vi "SSD1306_SaveFonts2File.vi"(1 "vi name":string) -> (0 "file name":string)   [LabVIEW 2014, in "QwaveSys_Interface.lvlib"]
uses:
  QwaveSys_Interface.lvlib
  <vilib>/Utility/traverseref.llb/TRef TravTarget.ctl
  <vilib>/Utility/sysdir.llb/System Directory Type.ctl
  <vilib>/Utility/traverseref.llb/VI Scripting - Traverse.lvlib
panel:
  out "error out":errorcluster
  out "found":bool
  out "Fonts":string
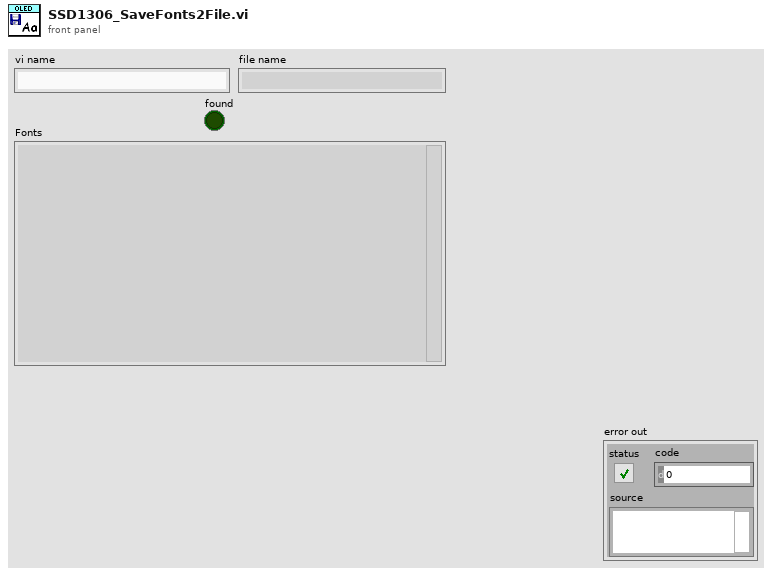
[diagram p1: front panel]
types:
  T1 = typedef "System Directory Type.ctl" = i32
  T2 = typedef "TRef TravTarget.ctl" = enum16{"FP", "BD", "Other"}
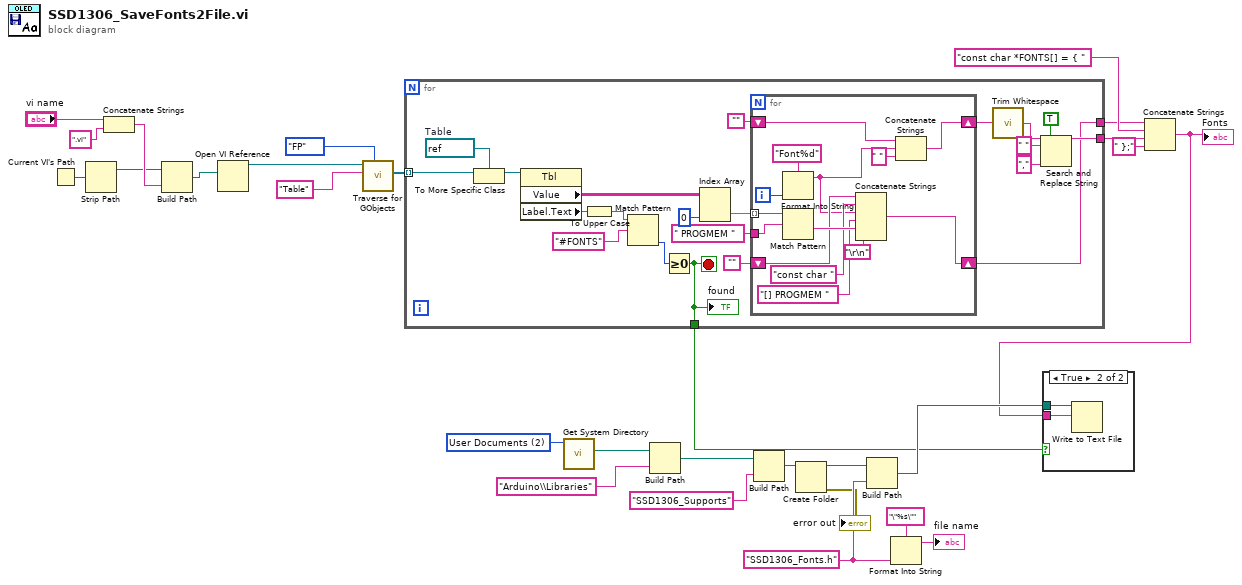
[diagram p0: block diagram]
diagram:
  w18 = T1 2 items=["User Home"=0, "User Desktop"=1, "User Documents"=2, "User Application Data"=3, "User Preferences"=4, "User Temporary"=5, "Public Documents"=6, "Public Application Data"=7, "Public Preferences"=8, "Public Cache"=13, "System Core Libraries"=9, "System Installed Libraries"=10, "Application Files"=11, "Boot Volume Root"=12] ("system directory type")
  w13 = "SSD1306_Fonts.h" ("string")
  n1 = Current VI's Path() -> (path=w22:path)
  n2 = Strip Path(path=w22) -> (stripped path=w21:path)  [unwired: 1 out]
  n3 = Concatenate Strings("vi name", ".vi" ("string")) -> (w23:string)
  n4 = Build Path(base path=w21, name or relative path=w23) -> (appended path=w19:path)
  n5 = Open VI Reference(vi path=w19) -> (vi reference=w28:refnum<vi>)  [unwired: 5 in, 1 out]
  n6 = call <vilib>:"Traverse for GObjects.vi"("Traverse Target"=TRef_TravTarget."FP", "Class Name"="Table", "VI Refnum"=w28) -> ("References"=w26:refnum<vi>[])  [unwired: 5 in, 3 out]
  n7 = for {
    tunnel: w26 -> [w48] mode=indexing
    tunnel: [w37] -> w8
    tunnel: [w31] -> w6
    tunnel: [w29] -> w3
    stop <- w37 stop-if-true
    w47 = refnum<vi> refnum  # Table
    n8 = To More Specific Class(target class=w47, reference=w48) -> (specific class reference=w49:refnum<vi>)  [unwired: 1 in, 1 out]
    n9 = property class="Tbl"(reference=w49) -> ("Value"=w42:string[][], "Label.Text"=w46:string)  [unwired: 1 in, 2 out]
    n10 = To Upper Case(1:w46) -> (0:w45:string)
    n11 = Match Pattern(string=w45, regular expression="#FONTS") -> (offset past match=w44:i32)  [unwired: 1 in, 3 out]
    n12 = Greater Or Equal To 0?(x=w44) -> (x >= 0?=w37:bool)
    "found" <- w37
    n13 = Index Array(array=w42, index (col)=0 ("disabled index (col)")) -> (element=w40:string[])  [unwired: 1 in]
    n14 = for {
      tunnel: w40 -> [w63] mode=indexing
      tunnel: " PROGMEM " -> [w62]
      shift-right: [w54] -> w29
      shift-left: "" -> [w57]
      shift-right: [w50] -> w35
      shift-left: "" -> [w53]
      i -> [w61]
      n15 = Format Into String(format string="Font%d", w61) -> (resulting string=w52:string)  [unwired: 2 in, 1 out]
      n16 = Match Pattern(string=w63, regular expression=w62) -> (after substring=w60:string)  [unwired: 1 in, 3 out]
      n17 = Concatenate Strings(w57, "const char " ("format string"), w52, "[] PROGMEM " ("format string"), w60, "\r\n") -> (w54:string)
      n18 = Concatenate Strings(w53, w52, " " ("string")) -> (w50:string)
    }
    n19 = call <vilib>:"Trim Whitespace.vi"("string"=w35) -> ("trimmed string"=w34:string)  [unwired: 1 in]
    n20 = Search and Replace String(replace all?=TRUE ("replace all? (F)"), input string=w34, search string=" ", replace string="," ("replace string (\"\")")) -> (result string=w31:string)  [unwired: 4 in, 3 out]
  }
  n21 = call <vilib>:"Get System Directory.vi"("system directory type"=w18) -> ("system directory"=w16:path)  [unwired: 10 in]
  n22 = Build Path(base path=w16, name or relative path="Arduino\\Libraries") -> (appended path=w9:path)
  n23 = Build Path(base path=w9, name or relative path="SSD1306_Supports") -> (appended path=w12:path)
  n24 = Create Folder(path (use dialog)=w12) -> (created path=w11:path, error out=→"error out":errorcluster)  [unwired: 2 in, 1 out]
  n25 = Build Path(base path=w11, name or relative path=w13) -> (appended path=w10:path)
  n26 = Format Into String(format string="\"%s\"", w13) -> (resulting string=→"file name":string)  [unwired: 2 in, 1 out]
  n27 = Concatenate Strings(w3, "const char *FONTS[] = { " ("string"), w6, " };" ("string")) -> (w2:string)
  "Fonts" <- w2
  n28 = case shown="True" w8 {
    tunnel: w2 -> [_ w65]
    tunnel: w10 -> [_ w64]
    frame False {
    }
    frame True {
      n29 = Write to Text File(file (use dialog)=w64, text=w65) -> ()  [unwired: 2 in, 3 out]
    }
  }
